vi "3.7-UDP What Server.vi"() -> ()   [LabVIEW 2010]
doc: "Creates a named service and listens on the first available port. Whenever a client connects to the service, it responds with a message containing joystick data. The VI can be stopped using the STOP button."
uses:
  3.3-What/_typedefs/3.3-What Sensor Typedef.ctl
  3.3-What/_typedefs/3.3.1-LIDAR Data Typedef.ctl
  3.0-Global.vi
panel:
  out "4.3-What's Around Me? Sensor 2":T1
  in  "error in":errorcluster
  in  "stop":bool
  out "error out":errorcluster
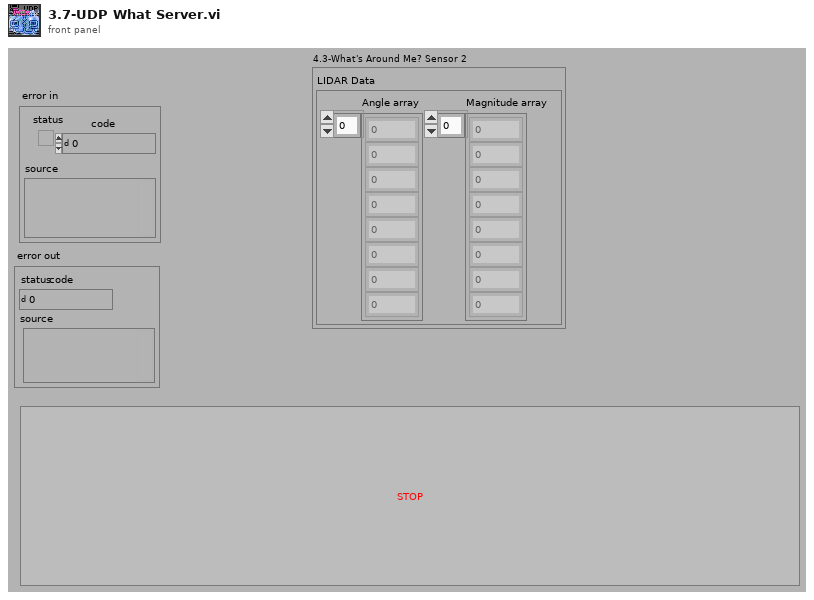
[diagram p1: front panel]
types:
  T1 = typedef "3.3-What Sensor Typedef.ctl" = cluster{"LIDAR Data":T2}
  T2 = typedef "3.3.1-LIDAR Data Typedef.ctl" = cluster{"Angle array":dbl[], "Magnitude array ":dbl[]}
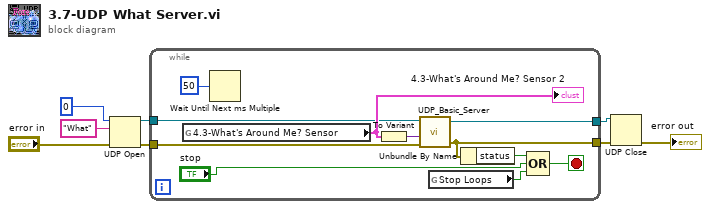
[diagram p0: block diagram]
diagram:
  n1 = UDP Open(8:"error in", 10:"What", 11:u16 0 ("port")) -> (port=w3:refnum<k16>, 0:w4:errorcluster)  [unwired: 2 in, 1 out]
  n2 = while {
    tunnel: w3 -> [w10]
    tunnel: w4 -> [w12]
    tunnel: [w11] -> w2
    tunnel: [w9] -> w1
    stop <- w19 stop-if-true
    n3 = global read "3.0-Global.vi" "4.3-What's Around Me? Sensor"() -> (w13:T1)
    "4.3-What's Around Me? Sensor 2" <- w13
    n4 = Wait Until Next ms Multiple(millisecond multiple=u32 50) -> ()  [unwired: 1 out]
    n5 = To Variant(anything=w13) -> (Variant=w14:variant)
    n6 = call "UDP_Basic_Server.vi"("error In"=w12, "Data in"=w14, "Connection ID"=w10) -> ("warning out"=w11:errorcluster, "Connection ID out"=w9:refnum<k16>)  [unwired: 1 in, 1 out]
    n7 = global read "3.0-Global.vi" "Stop Loops"() -> (w16:bool)
    n8 = Unbundle By Name(w11) -> ("status"=w15:bool)
    n9 = Compound Arithmetic op=OR(w15, "stop", w16) -> (w19:bool)
  }
  n10 = UDP Close(connection ID=w1, 8:w2) -> (error out=→"error out":errorcluster)  [unwired: 1 out]
